vi "MU Calc PRES_POS.vi"(7 "writeVerify":u32, 8 "error in (no error)":errorcluster, 10 "value":u64, 11 "handle":u64) -> (0 "error out (no error)":errorcluster)   [LabVIEW 2017, in "MU_3SL_interface.lvlib"]
uses:
  MU_3SL_interface.lvlib
  lib/MU_3SL_interface.dll
panel:
  out "function return":u32
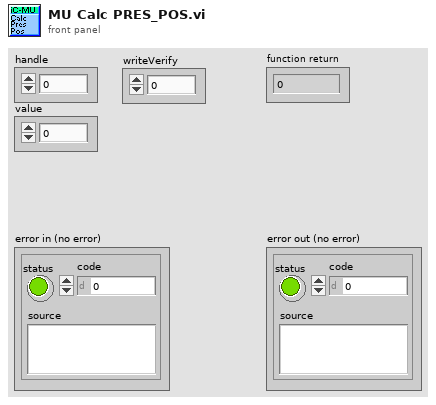
[diagram p1: front panel]
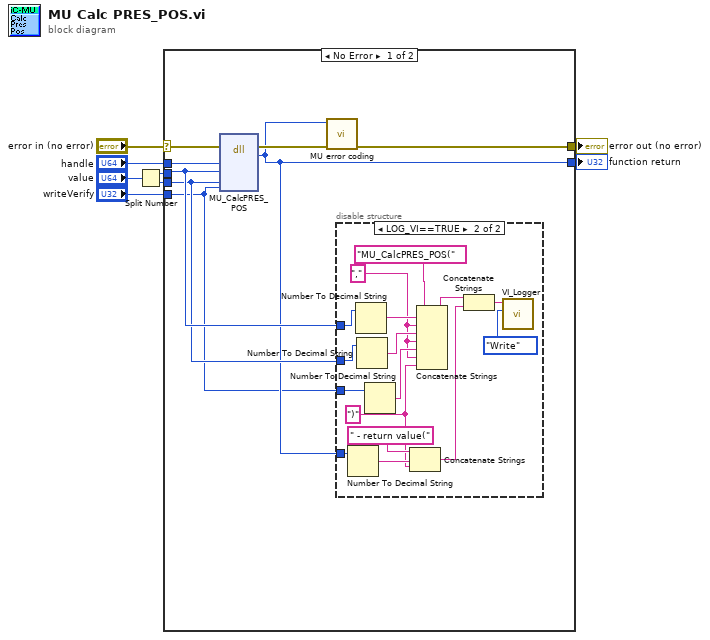
[diagram p0: block diagram]
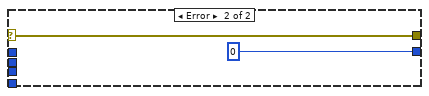
[diagram p3: hidden frame]
diagram:
  n1 = Split Number(x="value") -> (hi(x)=w2:u32, lo(x)=w1:u32)
  n2 = case shown="No Error" "error in (no error)" {
    selector: "error in (no error)" -> [w13 w34]
    tunnel: [w10 u32 0] -> w8
    tunnel: "handle" -> [w16 _]
    tunnel: [w14 w34] -> w6
    tunnel: w2 -> [w12 _]
    tunnel: "writeVerify" -> [w9 _]
    tunnel: w1 -> [w11 _]
    frame No Error {
      n3 = dll-call lib="C:/Users/bes/AppData/Roaming/work/mu_9so/icsubmodules/soft_mu_3sl_master/lv_interface/lib/MU_3SL_interface**.*" fn="MU_CalcPRES_POS"(error in=w13, "handle"=w16, "valueHigh"=w12, "valueLow"=w11, "writeVerify"=w9) -> (error out=w15:errorcluster, "return type"=w10:u32)  [unwired: 6 in, 1 out]
      n4 = call "MU error coding.vi"("error in (no error)"=w15, "function return in"=w10) -> ("error out"=w14:errorcluster)  [unwired: 9 in]
      n5 = disable-structure shown="LOG_VI==TRUE" {
        disable-tunnel: w10 -> [_ w30]
        disable-tunnel: w12 -> [_ w25]
        disable-tunnel: w11 -> [_ w23]
        disable-tunnel: w9 -> [_ w20]
        frame condition #0 {
        }
        frame condition #1 (active) {
          w19 = ")" ("string")
          w17 = "," ("string")
          n6 = Number To Decimal String(number=w30) -> (decimal integer string=w29:string)  [unwired: 1 in]
          n7 = Number To Decimal String(number=w25) -> (decimal integer string=w24:string)  [unwired: 1 in]
          n8 = Number To Decimal String(number=w23) -> (decimal integer string=w22:string)  [unwired: 1 in]
          n9 = Number To Decimal String(number=w20) -> (decimal integer string=w18:string)  [unwired: 1 in]
          n10 = Concatenate Strings(" - return value(" ("string"), w29, w19) -> (w27:string)
          n11 = Concatenate Strings("MU_CalcPRES_POS(" ("Info in"), w24, w17, w22, w17, w18, w17, w19) -> (w28:string)
          n12 = Concatenate Strings(w28, w27) -> (w26:string)
          n13 = call "VI_Logger.vi"("Action (Read)"=enum16{"Write", "Read"}."Write", "Info in"=w26) -> ()  [unwired: 8 in, 2 out]
        }
      }
    }
    frame Error {
    }
  }
  "function return" <- w8
  "error out (no error)" <- w6
